vi "WaitingForAck.vi"(11 "BaseDriver in":refnum<class "BaseDriver.lvclass">) -> (0 "Time left":u32, 1 "Timed out?":bool, 2 "Waiting?":bool, 3 "BaseDriver out":refnum<class "BaseDriver.lvclass">)   [LabVIEW 2013, in "BaseDriver.lvclass"]
doc: "Returns the state of the driver, if it is wating for a response from the remote destination and/or if the expected response has timed out"
uses:
  BaseDriver.lvclass
  BaseDriver.lvclass/BaseDriver.ctl
  Message/BaseMessage/BaseMessage.lvclass/BaseMessage.ctl
  driver_state.ctl
  Message/BaseMessage/Read Timeout.vi
  Message/BaseMessage/BaseMessage.lvclass
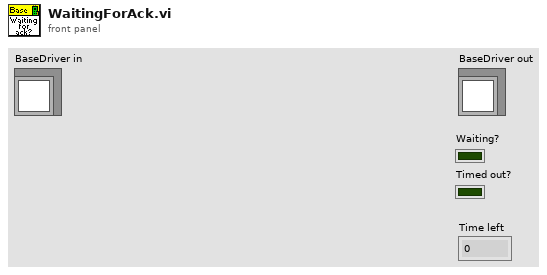
[diagram p1: front panel]
types:
  T1 = typedef "driver_state.ctl" = enum16{"Idle", "Wait for ack"}
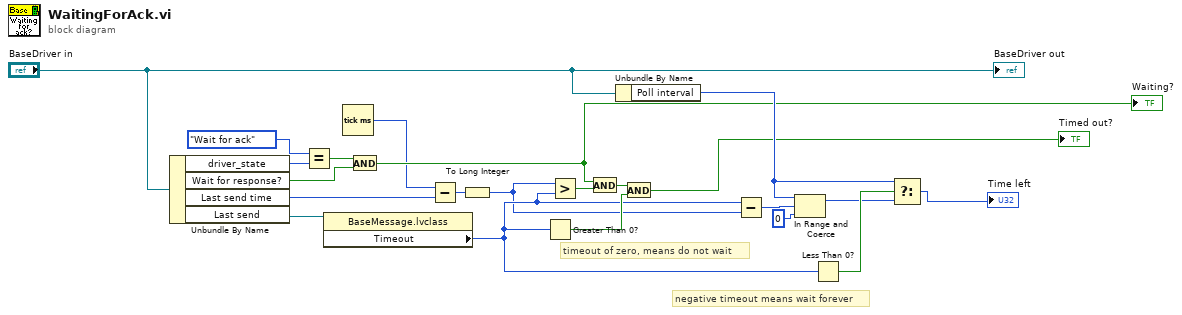
[diagram p0: block diagram]
diagram:
  # "timeout of zero, means do not wait"
  # "negative timeout means wait forever"
  n1 = Unbundle By Name("BaseDriver in") -> ("driver_state"=w21:T1, "Wait for response?"=w17:bool, "Last send time"=w8:u32, "Last send"=w22:refnum<class "BaseMessage.lvclass">)
  n2 = Equal?(x=driver_state."Wait for ack", y=w21) -> (x = y?=w18:bool)
  n3 = property on="Property Node" class="BaseMessage.lvclass"(reference=w22) -> ("Timeout"=w6:i32)  [unwired: 1 in, 2 out]
  n4 = Tick Count (ms)() -> (millisecond timer value=w1:u32)
  n5 = And(x=w18, y=w17) -> (x .and. y?=w3:bool)
  "Waiting?" <- w3
  n6 = Subtract(x=w1, y=w8) -> (x-y=w7:u32)
  n7 = To Long Integer(number=w7) -> (32bit integer=w5:i32)
  n8 = Greater Than 0?(x=w6) -> (x > 0?=w15:bool)
  n9 = Greater?(x=w5, y=w6) -> (0:w19:bool)
  n10 = And(x=w3, y=w19) -> (x .and. y?=w16:bool)
  n11 = Unbundle By Name("BaseDriver in") -> ("Poll interval"=w9:i32)
  n12 = And(x=w16, y=w15) -> (x .and. y?=→"Timed out?":bool)
  n13 = Subtract(x=w6, y=w5) -> (x-y=w14:i32)
  n14 = In Range and Coerce(upper limit=w9, x=w14, lower limit=0) -> (coerced(x)=w11:i32)  [unwired: 1 out]
  n15 = Less Than 0?(x=w6) -> (x < 0?=w12:bool)
  n16 = Select(t=w9, s=w12, f=w11) -> (s? t:f=→"Time left":i32)
  "BaseDriver out" <- "BaseDriver in"
